vi "_Split_DB_Read.vi"(0 "Lists of S7 Read Items":T1[](array[typedef]) {"Address Areas" items=["I/O (P)"=128, "Input (I)"=129, "Output (Q)"=130, "Bit Memory (M)"=131, "Data (DB)"=132, "Instance Data (DI)"=133, "Local Data (L)"=134, "Predecessor Local Data (VL)"=135]; "Read / Write" items=["Read"=4, "Write"=5]; "Bit Number / Byte Length" max=7 step=1}, 1 "Max Size":u8=222, 3 "S7 Read Array Input":T1[](array[typedef]) {"Address Areas" items=["I/O (P)"=128, "Input (I)"=129, "Output (Q)"=130, "Bit Memory (M)"=131, "Data (DB)"=132, "Instance Data (DI)"=133, "Local Data (L)"=134, "Predecessor Local Data (VL)"=135]; "Read / Write" items=["Read"=4, "Write"=5]; "Bit Number / Byte Length" max=7 step=1}) -> (5 "Optimized S7 Read Array Output":T1[](array[typedef]) {"Address Areas" items=["I/O (P)"=128, "Input (I)"=129, "Output (Q)"=130, "Bit Memory (M)"=131, "Data (DB)"=132, "Instance Data (DI)"=133, "Local Data (L)"=134, "Predecessor Local Data (VL)"=135]; "Read / Write" items=["Read"=4, "Write"=5]; "Bit Number / Byte Length" max=7 step=1})   [LabVIEW 2017, in "S7 TCP.lvlib"]
uses:
  S7 TCP.lvlib
  S7 Read Write Cluster.ctl
  Data Type.ctl
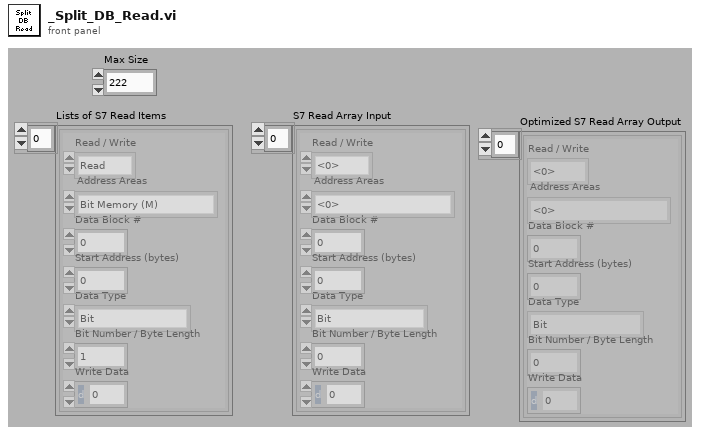
[diagram p1: front panel]
types:
  T1 = typedef "S7 TCP.lvlib/S7 Read Write Cluster.ctl" = cluster{"Read / Write":u8, "Address Areas":u8, "Data Block #":u16, "Start Address (bytes)":u32, "Data Type":T2, "Bit Number / Byte Length":u8, "Write Data":dbl}
  T2 = typedef "S7 TCP.lvlib/Data Type.ctl" = enum16{"Bit", "Byte (U8)", "Signed Byte (I8)", "Word (U16)", "Signed Word (I16)", "Long (U32)", "Signed Long (I32)", "Real (SGL)", "Defined Byte Length"}
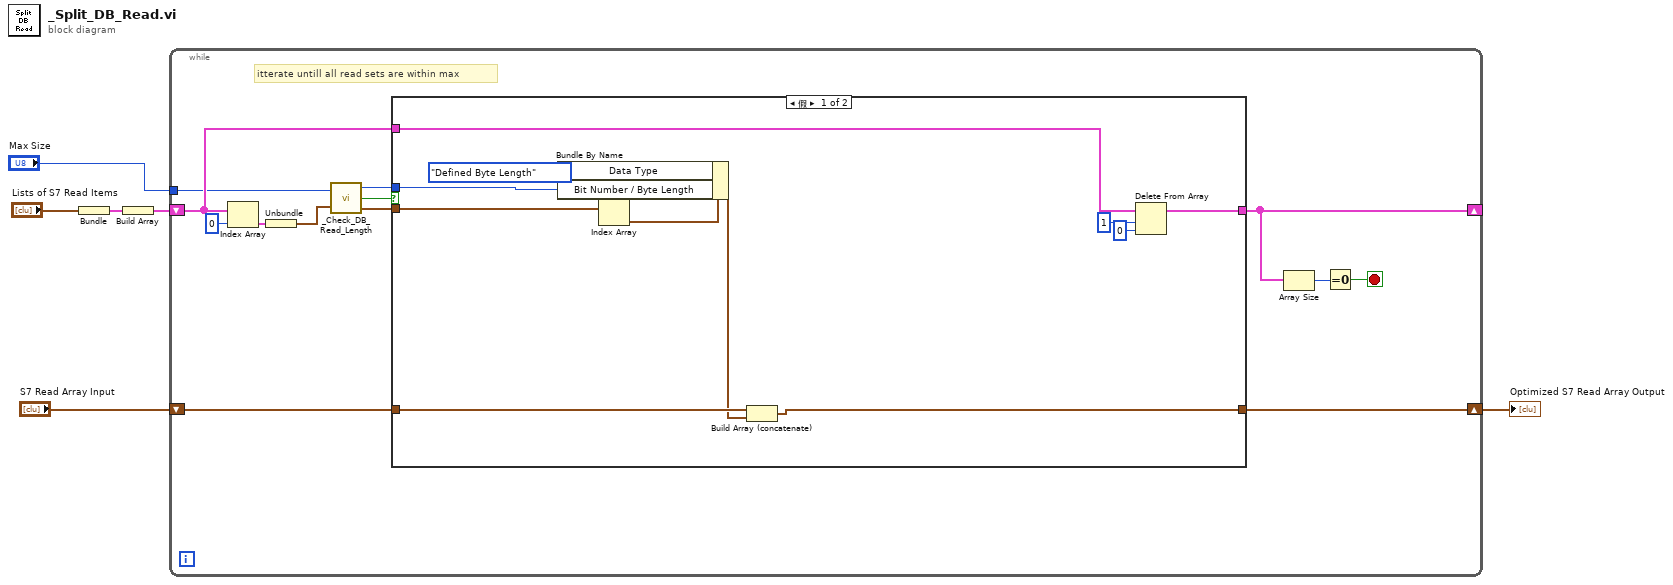
[diagram p0: block diagram]
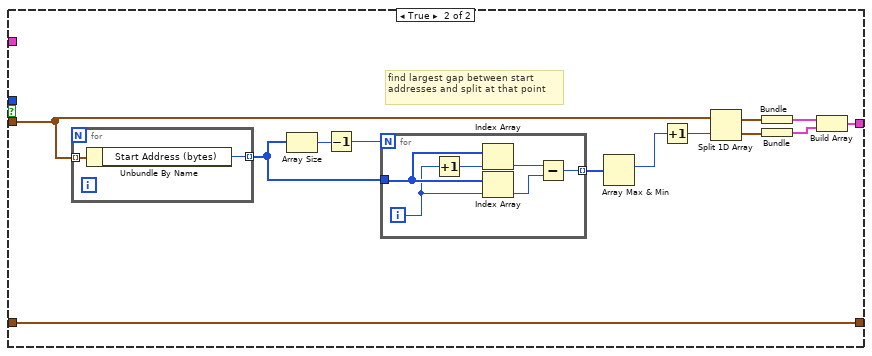
[diagram p2: hidden frame]
diagram:
  n1 = Bundle("Lists of S7 Read Items"="Lists of S7 Read Items") -> (w2:cluster{"Lists of S7 Read Items":T1[]})  [unwired: 1 in]
  n2 = Build Array(w2) -> (w1:cluster{"Lists of S7 Read Items":T1[]}[])
  n3 = while {
    shift-right: [w8] -> _
    shift-left: w1 -> [w15]
    shift-right: [w13] -> w5
    shift-left: "S7 Read Array Input" -> [w19]
    tunnel: "Max Size" -> [w11]
    stop <- w10 stop-if-true
    # "itterate untill all read sets are within max"
    n4 = Index Array(array=w15, index=0 ("index (row)")) -> (element=w12:cluster{"Lists of S7 Read Items":T1[]})
    n5 = Unbundle(w12) -> ("Lists of S7 Read Items"=w9:T1[])
    n6 = call "_Check_DB_Read_Length.vi"("Max Size"=w11, "List of S7 Read Items"=w9) -> ("Byte Length"=w16:u32, "Too Long?"=w17:bool, "Sorted List of S7 Read Items"=w18:T1[])
    n7 = case shown="假" w17 {
      tunnel: w19 -> [w30 w43]
      tunnel: [w29 w43] -> w13
      tunnel: w18 -> [w26 w36]
      tunnel: w16 -> [w25 _]
      tunnel: [w23 w31] -> w8
      tunnel: w15 -> [w24 _]
      frame False {
        n8 = Index Array(array=w26) -> (element=w28:T1)  [unwired: 1 in]
        n9 = Bundle By Name(cluster=w28, "Data Type"=Data_Type."Defined Byte Length", "Bit Number / Byte Length"=w25) -> (w27:T1)
        n10 = Build Array (concatenate)(w30, w27) -> (w29:T1[])
        n11 = Delete From Array(array=w24, length=1, index=0 ("index (row)")) -> (array with subset deleted=w23:cluster{"Lists of S7 Read Items":T1[]}[])  [unwired: 1 out]
      }
      frame True {
        # "find largest gap between start addresses and split at that point"
        n12 = for {
          tunnel: w36 -> [w45] mode=indexing
          tunnel: [w44] -> w41 mode=indexing
          n13 = Unbundle By Name(w45) -> ("Start Address (bytes)"=w44:u32)
        }
        n14 = Array Size(array=w41) -> (size(s)=w38:i32)
        n15 = Decrement(x=w38) -> (x-1=w37:i32)
        n16 = for {
          N: w37 -> [_]
          tunnel: w41 -> [w51]
          tunnel: [w46] -> w39 mode=indexing
          i -> [w50]
          n17 = Increment(x=w50) -> (x+1=w49:i32)
          n18 = Index Array(array=w51, index=w49) -> (element=w48:u32)
          n19 = Index Array(array=w51, index=w50) -> (element=w47:u32)
          n20 = Subtract(x=w48, y=w47) -> (x-y=w46:u32)
        }
        n21 = Array Max & Min(array=w39) -> (max index (indices)=w40:i32)  [unwired: 3 out]
        n22 = Increment(x=w40) -> (x+1=w42:i32)
        n23 = Split 1D Array(array=w36, index=w42) -> (first subarray=w35:T1[], second subarray=w33:T1[])
        n24 = Bundle(w35) -> (w34:cluster{T1[]})  [unwired: 1 in]
        n25 = Bundle(w33) -> (w32:cluster{T1[]})  [unwired: 1 in]
        n26 = Build Array(w34, w32) -> (w31:cluster{T1[]}[])
      }
    }
    n27 = Array Size(array=w8) -> (size(s)=w7:i32)
    n28 = Equal To 0?(x=w7) -> (x = 0?=w10:bool)
  }
  "Optimized S7 Read Array Output" <- w5
